vi "Test-AggregationLifetimeError.vi"() -> ()   [LabVIEW 2013]
uses:
  src/SMO/SMO.lvclass
panel:
  out "error out":errorcluster
  out "Can't be stopped":bool
  # "<< Error 1556 illustrates a bug with version 1.1.7.31 \n\n(Essentially because B is destroyed by top-level before A is stopped, and A depends on B that no longer exists on stopping... this error should be handled by framework. Reverse the launching order to demonstrate bug is lifetime-related)"
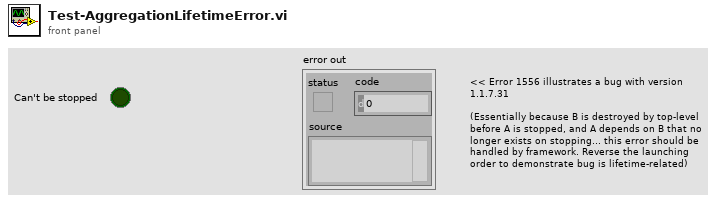
[diagram p1: front panel]
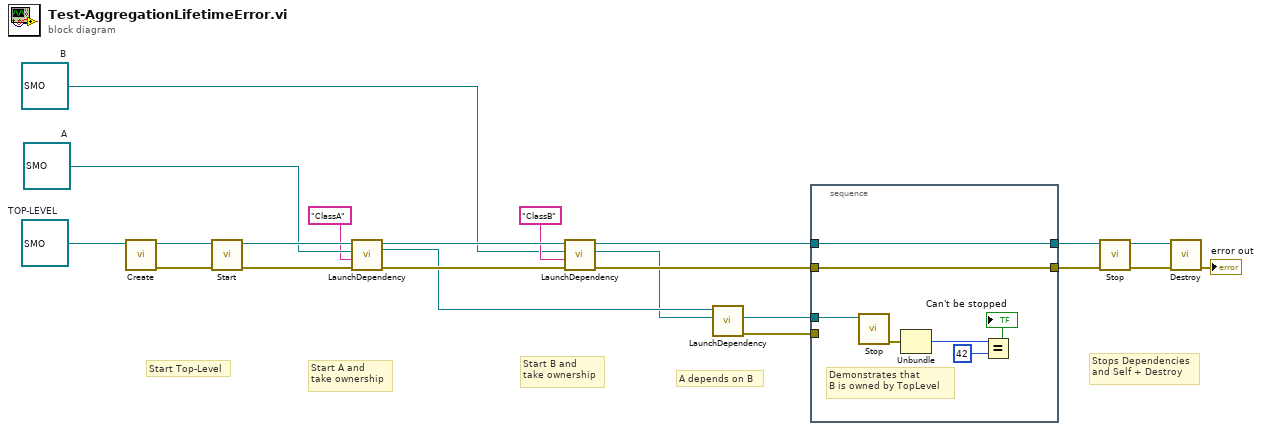
[diagram p0: block diagram]
diagram:
  w15 = refnum<class "SMO.lvclass"> refnum  # B
  w19 = refnum<class "SMO.lvclass"> refnum  # A
  w22 = refnum<class "SMO.lvclass"> refnum  # TOP-LEVEL
  # "Stops Dependencies\nand Self + Destroy"
  # "A depends on B"
  # "Start B and\ntake ownership"
  # "Start A and\ntake ownership"
  # "Start Top-Level"
  n1 = call "Create.vi"("SMO"=w22) -> ("error out"=w13:errorcluster, "SMO out"=w21:refnum<class "SMO.lvclass">)  [unwired: 8 in, 1 out]
  n2 = call "Start.vi"("error in (no error)"=w13, "SMO"=w21) -> ("error out"=w14:errorcluster, "SMO out"=w20:refnum<class "SMO.lvclass">)  [unwired: 8 in]
  n3 = call "LaunchDependency.vi"("error in (no error)"=w14, "Dependency Name"="ClassA", "Dependency Type"=w19, "SMO in"=w20) -> ("error out"=w12:errorcluster, "Dependency Reference"=w3:refnum<class "SMO.lvclass">, "SMO out"=w17:refnum<class "SMO.lvclass">)  [unwired: 4 in, 1 out]
  n4 = call "LaunchDependency.vi"("error in (no error)"=w12, "Dependency Name"="ClassB", "Dependency Type"=w15, "SMO in"=w17) -> ("error out"=w9:errorcluster, "Dependency Reference"=w2:refnum<class "SMO.lvclass">, "SMO out"=w10:refnum<class "SMO.lvclass">)  [unwired: 4 in, 1 out]
  n5 = call "LaunchDependency.vi"("Dependency Type"=w2, "SMO in"=w3) -> ("error out"=w11:errorcluster, "Dependency Reference"=w8:refnum<class "SMO.lvclass">)  [unwired: 6 in, 2 out]
  n6 = stacked-sequence {
    tunnel: w11 -> [_]
    tunnel: w10 -> [w24]
    tunnel: w9 -> [w23]
    tunnel: w8 -> [w29]
    tunnel: [w24] -> w7
    tunnel: [w23] -> w6
    frame #0 {
      # "Demonstrates that\nB is owned by TopLevel"
      n7 = call "Stop.vi"("SMO"=w29) -> ("error out"=w28:errorcluster)  [unwired: 9 in, 1 out]
      n8 = Unbundle(w28) -> ("code"=w27:i32)  [unwired: 2 out]
      n9 = Equal?(x=w27, y=42) -> (x = y?=→"Can't be stopped":bool)
    }
  }
  n10 = call "Stop.vi"("error in (no error)"=w6, "SMO"=w7) -> ("error out"=w4:errorcluster, "SMO out"=w5:refnum<class "SMO.lvclass">)  [unwired: 8 in]
  n11 = call "Destroy.vi"("error in (no error)"=w4, "SMO"=w5) -> ("error out"=→"error out":errorcluster)  [unwired: 9 in]
